vi "MRC Initialize All.vi"() -> (0 "error out":errorcluster)   [LabVIEW 2026]
uses:
  MrcLib.dll
  MrcLib.lvlib
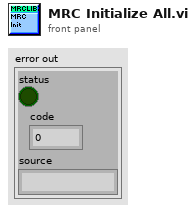
[diagram p1: front panel]
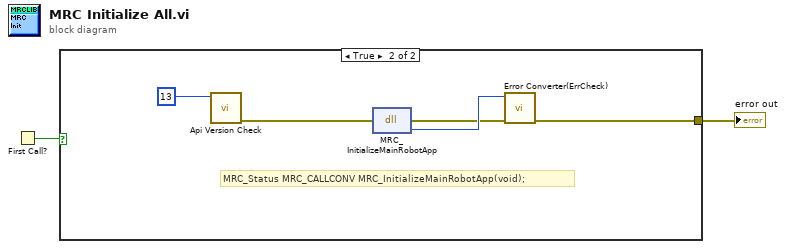
[diagram p0: block diagram]
diagram:
  n1 = First Call?() -> (First Call?: T/F=w2:bool)
  n2 = case shown="True" w2 {
    tunnel: [_ w5] -> w1
    frame False {
    }
    frame True {
      # "MRC_Status MRC_CALLCONV MRC_InitializeMainRobotApp(void);"
      n3 = call <vilib>:"Api Version Check.vi"("version"=u32 13) -> ("error out"=w3:errorcluster)  [unwired: 10 in]
      n4 = dll-call lib="MrcLib.*" fn="MRC_InitializeMainRobotApp"(error in=w3) -> (error out=w6:errorcluster, "return type"=w7:i32)  [unwired: 2 in, 1 out]
      n5 = call "Error Converter(ErrCheck).vi"("error in (no error)"=w6, "status"=w7) -> ("error out"=w5:errorcluster)  [unwired: 9 in]
    }
  }
  "error out" <- w1
